vi "Temperature Warning.vi"(9 "Threshold":dbl, 11 "Current Temperature":dbl) -> (2 "Threshold Exceeded?":bool)   [LabVIEW 2020]
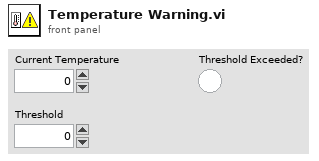
[diagram p1: front panel]
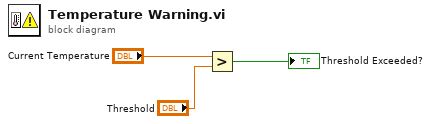
[diagram p0: block diagram]
diagram:
  n1 = Greater?(x="Current Temperature", y="Threshold") -> (0:→"Threshold Exceeded?":bool)
